vi "M14_IMU_Hardware_Begin.vi"   [LabVIEW 2019]
uses:
  <vilib>/Rock Robotics/WPI/ThirdParty/Phoenix-LabVIEW/Pigeon IMU/CTRE_PigeonIMU_Open_CAN.vi
  M14_IMU_Hardware_Globals.vi
types:
  T1 = typedef "CTRE_PigeonIMU_DeviceRef.ctl" = cluster{"DeviceStatus":errorcluster, "Device Number":u8, "Type":T2, "Device ID":u32, "Handle":u64, "UsageFrame":u32, "Library Path":path}
  T2 = typedef "CTRE_PigeonIMU_ConnectionType.ctl" = u32
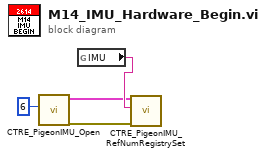
[diagram p0: block diagram]
diagram:
  n1 = call-poly <vilib>:"CTRE_PigeonIMU_Open.vi"("Device Number"=u8 6) -> ("error out"=w1:errorcluster, "PigeonIMUDevRef"=w3:T1)  [unwired: 9 in]
  n2 = global read "M14_IMU_Hardware_Globals.vi" "IMU"() -> (w4:string)
  n3 = call <vilib>:"CTRE_PigeonIMU_RefNumRegistrySet.vi"("error in (no error)"=w1, "refnum name"=w4, "PigeonIMUDevRef"=w3) -> ()  [unwired: 7 in, 2 out]
